vi "Nattify - Compute Top Row Vertical Delta.vi"(0 "controls":refnum<vi>[](array[refnum]), 5 "TermBnds[]":T1[](array[typedef]), 11 "error in":errorcluster) -> (4 "max vertical rectangle delta for controls from the top row":i16, 15 "error out":errorcluster)   [LabVIEW 2020]
uses:
  <vilib>/Utility/miscctls.llb/LVRectTypeDef.ctl
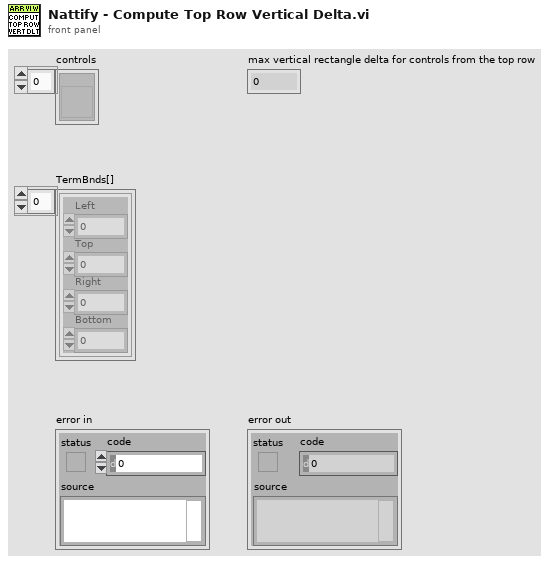
[diagram p1: front panel]
types:
  T1 = typedef "LVRectTypeDef.ctl" = cluster{"Left":i16, "Top":i16, "Right":i16, "Bottom":i16}
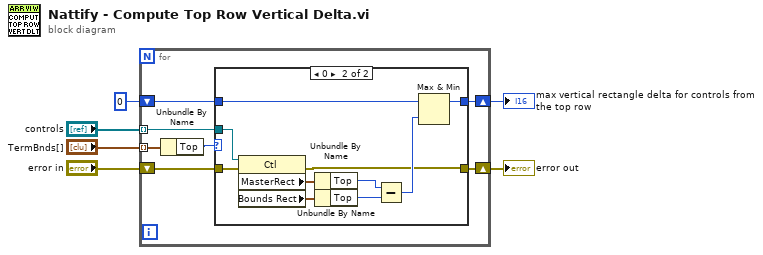
[diagram p0: block diagram]
diagram:
  n1 = for {
    tunnel: "controls" -> [w11] mode=indexing
    shift-right: [w7] -> w1
    shift-left: "error in" -> [w8]
    shift-right: [w13] -> w5
    shift-left: i16 0 -> [w12]
    tunnel: "TermBnds[]" -> [w10] mode=indexing
    n2 = Unbundle By Name(w10) -> ("Top"=w9:i16)
    n3 = case shown="0" w9 {
      tunnel: [w14 w25] -> w13
      tunnel: w12 -> [w14 w24]
      tunnel: w11 -> [_ w22]
      tunnel: w8 -> [w15 w21]
      tunnel: [w15 w16] -> w7
      frame Default {
      }
      frame 0 {
        n4 = property class="Ctl"(reference=w22, error in=w21) -> (error out=w16:errorcluster, "MasterRect"=w20:T1, "Bounds Rect"=w23:T1)  [unwired: 1 out]
        n5 = Unbundle By Name(w20) -> ("Top"=w19:i16)
        n6 = Unbundle By Name(w23) -> ("Top"=w18:i16)
        n7 = Subtract(x=w19, y=w18) -> (x-y=w17:i16)
        n8 = Max & Min(x=w24, y=w17) -> (max(x,y)=w25:i16)  [unwired: 1 out]
      }
    }
  }
  "max vertical rectangle delta for controls from the top row" <- w5
  "error out" <- w1
